vi "Run.vi"(8 "error in (no error)":errorcluster caption="entrée d'erreur (pas d'erreur)", 11 "Hastie_10_2.lvclass":refnum<class "Hastie_10_2.lvclass">) -> (0 "error out":errorcluster caption="sortie d'erreur", 2 "Data":T1, 3 "Hastie_10_2.lvclass":refnum<class "Hastie_10_2.lvclass">)   [LabVIEW 2020, in "Hastie_10_2.lvclass"]
doc: "Returns :\n\nX : array of shape [n_samples, 10]\n The input samples.\n\ny : array of shape [n_samples]\n The output values."
uses:
  Hastie_10_2.lvclass
  Hastie_10_2.lvclass/Hastie_10_2.ctl
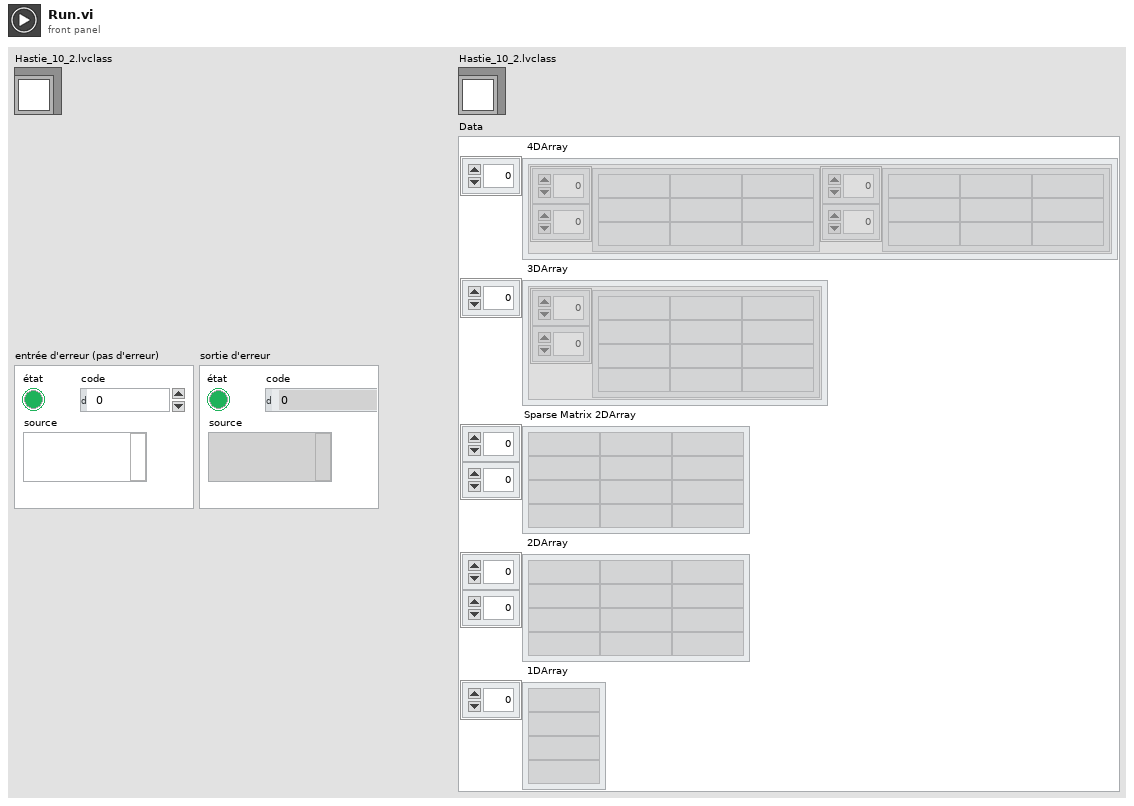
[diagram p1: front panel]
types:
  T1 = cluster{" 4DArray":cluster{"1":string[][], "2":string[][]}[], " 3DArray":cluster{"Tableau":string[][]}[], "Sparse Matrix 2DArray":string[][], " 2DArray":string[][], " 1DArray":string[]}
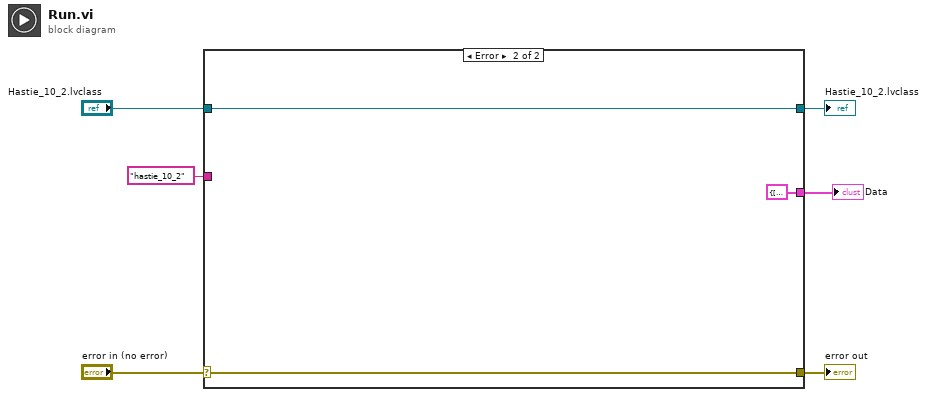
[diagram p0: block diagram]
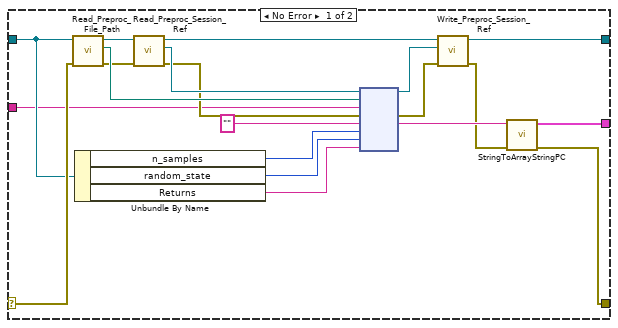
[diagram p2: hidden frame]
diagram:
  n1 = case shown="Error" "error in (no error)" {
    selector: "error in (no error)" -> [w15 w29]
    tunnel: [w8 w29] -> w5
    tunnel: [w11 w28] -> w3
    tunnel: "Hastie_10_2.lvclass" -> [w14 w28]
    tunnel: "hastie_10_2" -> [w13 _]
    tunnel: [w7 T1 {" 4DArray"=[], " 3DArray"=[], "Sparse Matrix 2DArray"=[], " 2DArray"=[], " 1DArray"=[]} ("Data")] -> w1
    frame No Error {
      n2 = call-dynamic "Read_Preproc_File_Path.vi"("error in (no error)"=w15, "Python in"=w14) -> ("error out"=w21:errorcluster, "File_Path"=w24:path, "Python out"=w26:refnum<class "Hastie_10_2.lvclass">)  [unwired: 7 in]
      n3 = Unbundle By Name(w14) -> ("n_samples"=w17:u32, "random_state"=w16:i32, "Returns"=w12:string)
      n4 = call-dynamic "Read_Preproc_Session_Ref.vi"("error in (no error)"=w21, "Python in"=w26) -> ("error out"=w22:errorcluster, "Session_ref"=w23:refnum<k35>, "Python out"=w25:refnum<class "Hastie_10_2.lvclass">)  [unwired: 7 in]
      n5 = node(w23, w24, w13, w22, "", w17, w16, w12) -> (w18:refnum<k35>, w20:errorcluster, w10:string)  [unwired: 3 in, 2 out]
      n6 = call-dynamic "Write_Preproc_Session_Ref.vi"("error in (no error)"=w20, "Session_ref"=w18, "Python in"=w25) -> ("error out"=w9:errorcluster, "Python out"=w11:refnum<class "Hastie_10_2.lvclass">)  [unwired: 7 in]
      n7 = call "StringToArrayStringPC.vi"("sortie d'erreur"=w9, "Return value"=w10) -> ("sortie d'erreur"=w8:errorcluster, "Data"=w7:T1)  [unwired: 8 in]
    }
    frame Error {
    }
  }
  "error out" <- w5
  "Hastie_10_2.lvclass" <- w3
  "Data" <- w1
